vi "Read Key.vi"   [LabVIEW 2020, in "NI_LVConfig.lvlib"]
doc: "Reads a value associated with a key in a specified section from the configuration data identified by <B>refnum</B>. If the key does not exist, the VI returns the default value. This VI supports multibyte characters in strings. Wire data to the <B>default value</B> input to determine the polymorphic instance to use or manually select the instance."
uses:
  <vilib>/Utility/config.llb/NI_LVConfig.lvlib
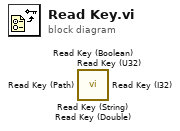
[diagram p0: block diagram]
diagram:
  n1 = call <vilib>:"Read Key (String).vi"() -> ()  [unwired: 8 in, 4 out]
  n2 = call <vilib>:"Read Key (U32).vi"() -> ()  [unwired: 8 in, 4 out]
  n3 = call <vilib>:"Read Key (Path).vi"() -> ()  [unwired: 8 in, 4 out]
  n4 = call <vilib>:"Read Key (I32).vi"() -> ()  [unwired: 8 in, 4 out]
  n5 = call <vilib>:"Read Key (Double).vi"() -> ()  [unwired: 8 in, 4 out]
  n6 = call <vilib>:"Read Key (Boolean).vi"() -> ()  [unwired: 8 in, 4 out]
